vi "Initialize Settings 1.0.vi"(8 "error in (no error)":errorcluster, 11 "settings 1.0":cluster{"key":string, "value":string}[](array[cluster])) -> (0 "error out":errorcluster, 3 "configuration 1.0":cluster{"name":string}={"name"="Transfer"})   [LabVIEW 2019, in "DSF Core.lvlib" / "Transfer Configuration.lvclass"]
uses:
  Transfer Configuration.lvclass
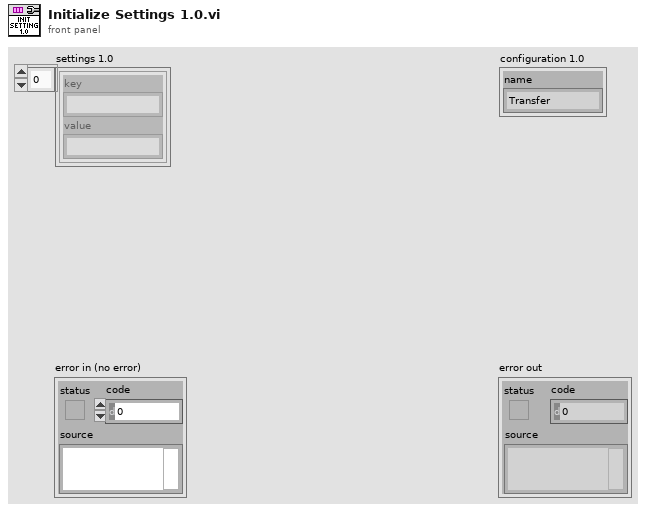
[diagram p1: front panel]
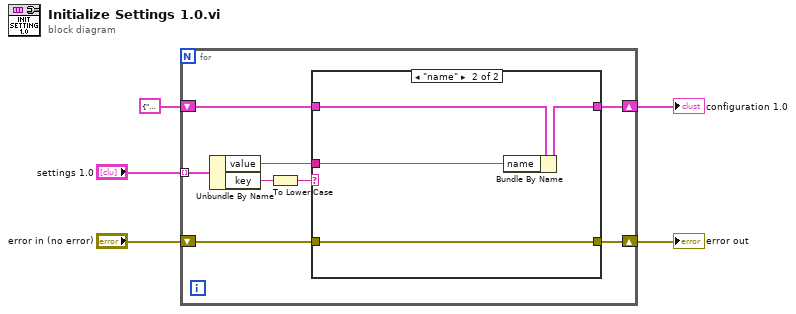
[diagram p0: block diagram]
diagram:
  n1 = for {
    shift-right: [w8] -> w1
    shift-left: cluster{"name":string} {"name"="Transfer"} ("configuration 1.0") -> [w9]
    tunnel: "settings 1.0" -> [w13] mode=indexing
    shift-right: [w6] -> w5
    shift-left: "error in (no error)" -> [w7]
    n2 = Unbundle By Name(w13) -> ("value"=w10:string, "key"=w12:string)
    n3 = To Lower Case(string=w12) -> (all lower case string=w11:string)
    n4 = case shown="\"name\"" w11 {
      tunnel: w10 -> [_ w16]
      tunnel: w9 -> [w15 w19]
      tunnel: [w15 w18] -> w8
      tunnel: w7 -> [w14 w17]
      tunnel: [w14 w17] -> w6
      frame Default {
        # "Unknown setting."
      }
      frame "name" {
        n5 = Bundle By Name(cluster=w19, "name"=w16) -> (w18:cluster{"name":string})
      }
    }
  }
  "error out" <- w5
  "configuration 1.0" <- w1
